vi "cycling structure demo Main.vi"() -> ()   [LabVIEW 2020]
doc: "This VI can be used as a launcher VI for the main application or as a debugging tool.\n_____\nBased on DQMH Project Template 6.1.0.94."
uses:
  Libraries/Rename As Application UI/cycling structure demo UI.lvlib
  Libraries/Launcher Support/Launcher Support.lvlib
  <vilib>/Peloton/Pelobuttons/Pelobuttons_lib_Pelobuttons.lvlib
  <vilib>/Peloton/Peloton Config/DCFG Framework/Peloton_lib_DCFG Framework.lvlib
  Libraries/Rename As Application Shared/Rename as Application Shared.lvlib
panel:
  in  "Config Views":string(combo)
  in  "Launch Peloton Config":bool
  in  "Launch UI API Tester":bool
  out "Command Line Arguments":string[](array[string])
  out "Module Running?":bool
  out "Status":string
  out "error out":errorcluster
  in  "Stop Module":bool
  in  "Start Module":bool
  # "See the Build_Final_EXE bookmarks on the diagram for instructions on using this VI as a launcher for an EXE."
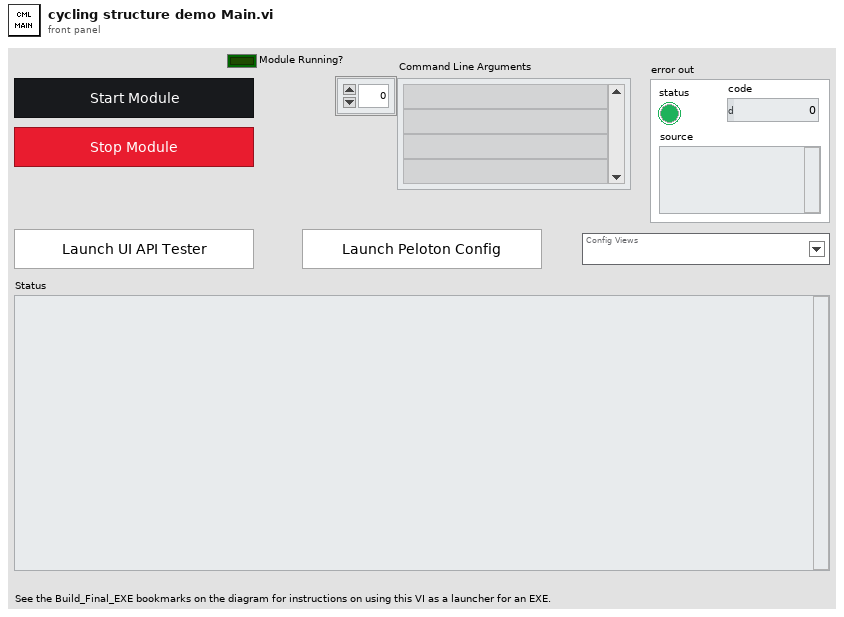
[diagram p1: front panel]
types:
  T1 = typedef "Peloton_lib_DCFG Framework.lvlib/Broadcast Events--cluster.ctl" = cluster{"Module Did Init":refnum<user-event>, "Status Updated":refnum<user-event>, "Error Reported":refnum<user-event>, "Module Did Stop":refnum<user-event>, "Update Module Execution Status":refnum<user-event>, "View Changed":refnum<user-event>, "Main Window Closed":refnum<user-event>, "Configuration Committed":refnum<user-event>, "Configuration Canceled":refnum<user-event>, "Views List Updated":refnum<user-event>, "Config Folder Path Updated":refnum<user-event>}
  T2 = typedef "cycling structure demo UI.lvlib/Broadcast Events--cluster.ctl" = cluster{"Module Did Init":refnum<user-event>, "Status Updated":refnum<user-event>, "Error Reported":refnum<user-event>, "Module Did Stop":refnum<user-event>, "Update Module Execution Status":refnum<user-event>}
  T3 = enum32{"invalid app kind", "Development System", "Run Time System", "Student Edition", "Embedded LabVIEW", "Evaluation", "Custom"}
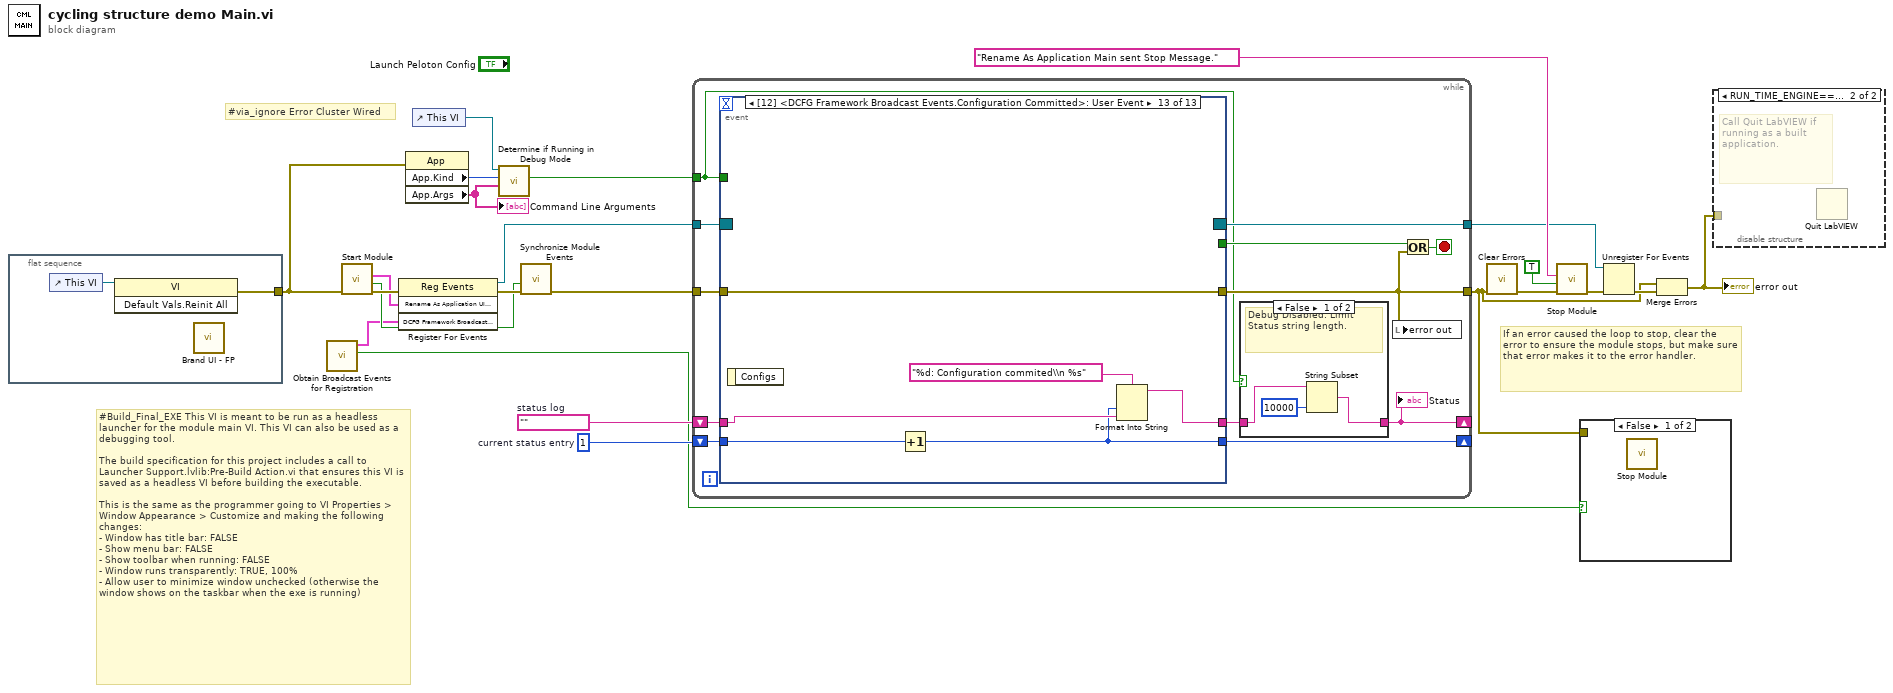
[diagram p0: block diagram]
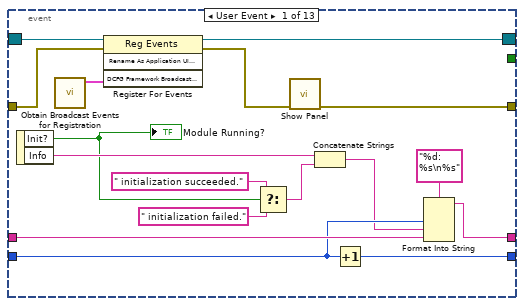
[diagram p4: hidden frame]
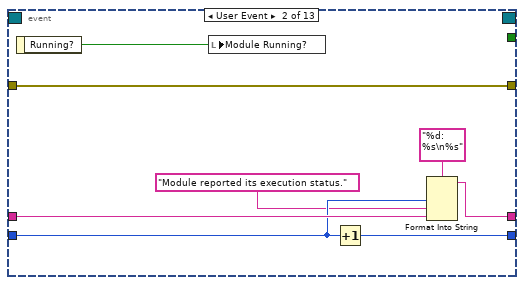
[diagram p5: hidden frame]
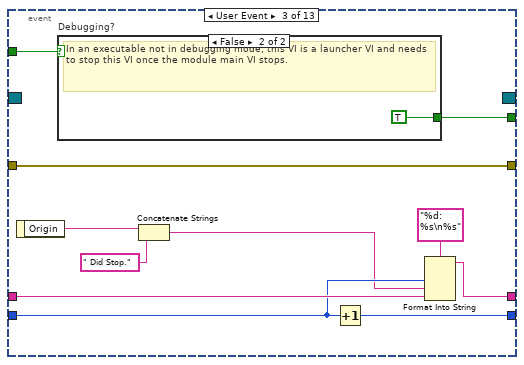
[diagram p6: hidden frame]
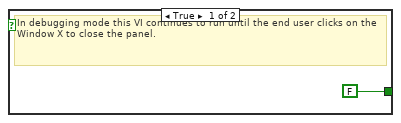
[diagram p7: hidden frame]
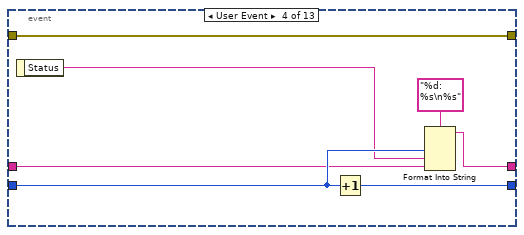
[diagram p8: hidden frame]
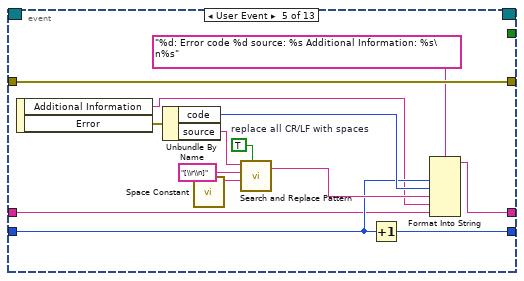
[diagram p9: hidden frame]
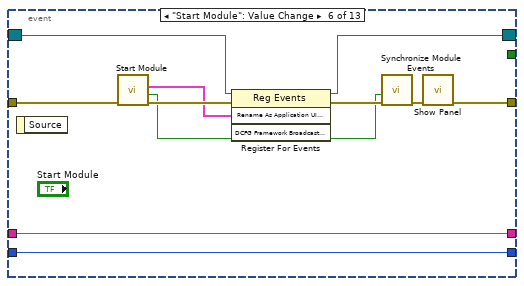
[diagram p10: hidden frame]
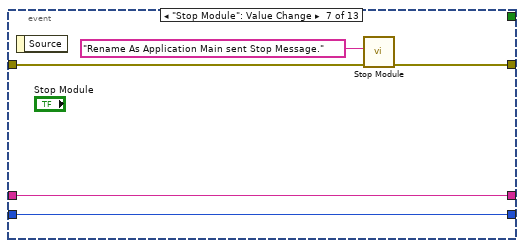
[diagram p11: hidden frame]
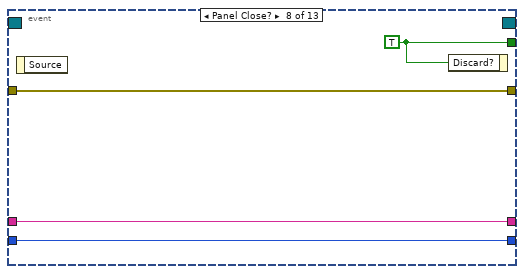
[diagram p12: hidden frame]
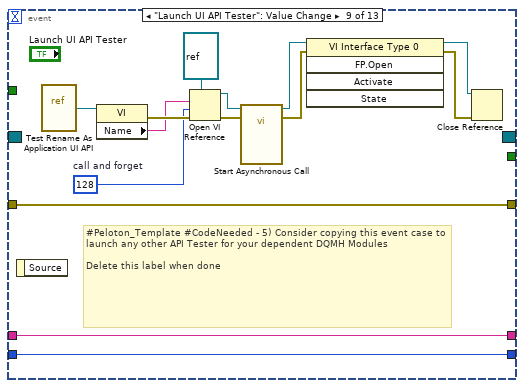
[diagram p13: hidden frame]
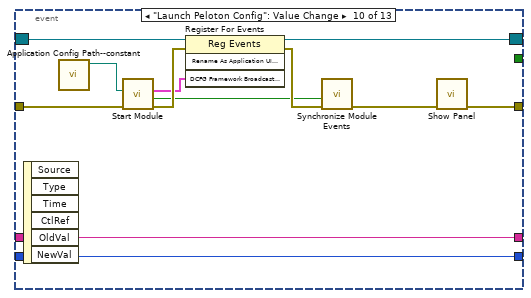
[diagram p14: hidden frame]
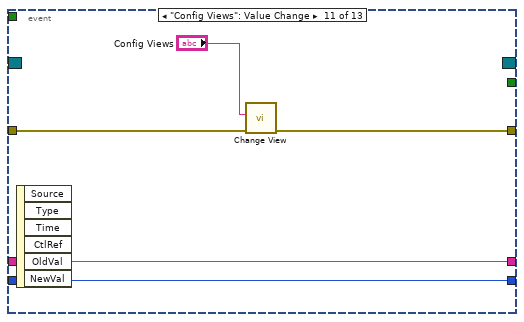
[diagram p15: hidden frame]
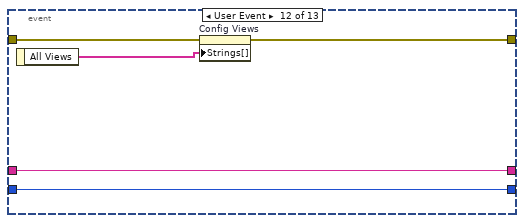
[diagram p16: hidden frame]
diagram:
  w12 = 1  # current status entry
  w13 = ""  # status log
  # "#via_ignore Error Cluster Wired"
  # "#Build_Final_EXE This VI is meant to be run as a headless launcher for the module main VI. This VI can also be used as a debugging tool. \n\nThe build specification for this project includes a call to Launcher Support.lvlib:Pre-Build Action.vi that ensures this VI is saved as a headless VI before building the executable.\n\nThis is the same as the programmer going to VI Properties > Window Appearance > Customize and making the following changes:\n- Window has title bar: FALSE\n- Show menu bar: FALSE\n- Show toolbar when running: FALSE\n- Window runs transparently: TRUE, 100%\n- Allow user to minimize window unchecked (otherwise the window shows on the taskbar when the exe is running)"
  # "If an error caused the loop to stop, clear the error to ensure the module stops, but make sure that error makes it to the error handler."
  n1 = flat-sequence {
    tunnel: [w25] -> w16
    frame #0 {
      n2 = control-ref of="This VI"() -> (w24:refnum<vi>)
      n3 = invoke on="Invoke Node" class="VI" method="Default Vals.Reinit All"(reference=w24) -> (error out=w25:errorcluster)  [unwired: 2 in, 2 out]
      n4 = call <vilib>:"Brand UI - FP.vi"() -> ()  [unwired: 12 in]
    }
  }
  n5 = call <vilib>:"Obtain Broadcast Events for Registration.vi"() -> ("Already running?"=w2:bool, "DCFG Framework Broadcast Events"=w1:T1)  [unwired: 9 in, 1 out]
  n6 = call <vilib>:"Start Module.vi"("error in"=w16) -> ("error out"=w19:errorcluster, "Wait for Event Sync?"=w9:bool, "Rename As Application UI Broadcast Events"=w8:T2)  [unwired: 7 in, 1 out]
  n7 = register-events(error in=w19, w8, w1) -> (reference out=w7:refnum<event-registration>, error out=w20:errorcluster)  [unwired: 1 in]
  n8 = property on="Property Node" class="App"(error in=w16) -> ("App.Kind"=w3:T3, "App.Args"=w6:string[])  [unwired: 1 in, 2 out]
  "Command Line Arguments" <- w6
  n9 = control-ref of="This VI"() -> (w5:refnum<vi>)
  n10 = call "Determine if Running in Debug Mode.vi"("App.Args"=w6, "App.Kind"=w3, "Launcher VI ref"=w5) -> ("Debug mode?"=w4:bool)  [unwired: 8 in]
  n11 = call <vilib>:"Synchronize Module Events.vi"("error in"=w20, "Wait for Event Sync?"=w9) -> ("error out"=w17:errorcluster)  [unwired: 9 in]
  n12 = while {
    tunnel: w7 -> [w35]
    tunnel: [w36] -> w15
    shift-right: [w27] -> _
    shift-left: w13 -> [w32]
    shift-right: [w31] -> _
    shift-left: w12 -> [w33]
    tunnel: w17 -> [w37]
    tunnel: [w29] -> w11
    tunnel: w4 -> [w26]
    stop <- w30 stop-if-true
    n13 = event shown="[12] <DCFG Framework Broadcast Events.Configuration Committed>: User Event" {
      selector: w35 -> [w44 _ _ _ _ w102 _ _ _ w139 _ _ _]
      dyn-events: [w43 _ _ _ _ w101 _ _ _ w138 _ _ _] -> w29
      timeout: _ -> [_ _ _ _ _ _ _ _ _ _ _ _ _]
      tunnel: [_ _ w68 _ _ _ _ w119 _ _ _ _ _] -> w34
      tunnel: [w57 w66 w77 w86 w100 w107 w116 w120 w134 w146 w150 w155 w162] -> w36
      tunnel: w33 -> [w53 w63 w74 w82 w90 w105 w113 w117 w128 w140 w148 w153 w159]
      tunnel: w32 -> [w54 w64 w75 w81 w88 w106 w114 w118 w129 w141 w149 w154 w160]
      tunnel: [w51 w61 w72 w83 w91 w106 w114 w118 w129 w141 w149 w154 w161] -> w28
      tunnel: [w52 w62 w73 w85 w89 w105 w113 w117 w128 w140 w148 w153 w158] -> w31
      tunnel: w37 -> [w58 w66 w77 w86 w100 w109 w115 w120 w134 w143 w151 w156 w162]
      tunnel: w26 -> [_ _ w67 _ _ _ _ _ _ _ _ _ _]
      event User Event {
        n14 = event-data() -> ("Init?"=w48:bool, "Info"=w50:string)  [unwired: 1 in]
        "Module Running?" <- w48
        n15 = call <vilib>:"Obtain Broadcast Events for Registration.vi"() -> ("DCFG Framework Broadcast Events"=w42:T1)  [unwired: 9 in, 2 out]
        n16 = register-events(reference=w44, error in=w58, w42) -> (reference out=w43:refnum<event-registration>, error out=w56:errorcluster)  [unwired: 1 in]
        n17 = Select(t=" initialization succeeded.", s=w48, f=" initialization failed.") -> (s? t:f=w45:string)
        n18 = call <vilib>:"Show Panel.vi"("error in (no error)"=w56) -> ("error out"=w57:errorcluster)  [unwired: 10 in]
        n19 = Concatenate Strings(w50, w45) -> (w49:string)
        n20 = Increment(x=w53) -> (x+1=w52:i32)
        n21 = Format Into String(format string="%d: %s\n%s", w53, w49, w54) -> (resulting string=w51:string)  [unwired: 2 in, 1 out]
      }
      event User Event {
        n22 = event-data() -> ("Running?"=w59:bool)  [unwired: 1 in]
        n23 = local write "Module Running?"(w59) -> ()
        n24 = Increment(x=w63) -> (x+1=w62:i32)
        n25 = Format Into String(format string="%d: %s\n%s", w63, "Module reported its execution status.", w64) -> (resulting string=w61:string)  [unwired: 2 in, 1 out]
      }
      event User Event {
        n26 = event-data() -> ("Origin"=w71:string)  [unwired: 1 in]
        n27 = case "Debugging?" shown="False" w67 {
          tunnel: [FALSE ("Discard?") TRUE ("Discard?")] -> w68
          frame True {
            # "In debugging mode this VI continues to run until the end user clicks on the Window X to close the panel."
          }
          frame False {
            # "In an executable not in debugging mode, this VI is a launcher VI and needs to stop this VI once the module main VI stops."
          }
        }
        n28 = Concatenate Strings(w71, " Did Stop.") -> (w70:string)
        n29 = Increment(x=w74) -> (x+1=w73:i32)
        n30 = Format Into String(format string="%d: %s\n%s", w74, w70, w75) -> (resulting string=w72:string)  [unwired: 2 in, 1 out]
      }
      event User Event {
        n31 = event-data() -> ("Status"=w80:string)  [unwired: 1 in]
        n32 = Increment(x=w82) -> (x+1=w85:i32)
        n33 = Format Into String(format string="%d: %s\n%s", w82, w80, w81) -> (resulting string=w83:string)  [unwired: 2 in, 1 out]
      }
      event User Event {
        w95 = TRUE  # replace all CR/LF with spaces
        n34 = event-data() -> ("Additional Information"=w87:string, "Error"=w99:errorcluster)  [unwired: 1 in]
        n35 = Unbundle By Name(w99) -> ("code"=w92:i32, "source"=w93:string)
        n36 = call <vilib>:"Space Constant.vi"() -> ("String"=w96:string)
        n37 = call <vilib>:"Search and Replace Pattern.vi"("string"=w93, "regular expression (\"\")"="[\\r\\n]" ("regular expression (\"\")"), "replace string (\"\")"=w96, "replace all? (F)"=w95) -> ("result string"=w94:string)  [unwired: 1 in, 1 out]
        n38 = Increment(x=w90) -> (x+1=w89:i32)
        n39 = Format Into String(format string="%d: Error code %d source: %s Additional Information: %s\n%s", w90, w92, w94, w87, w88) -> (resulting string=w91:string)  [unwired: 2 in, 1 out]
      }
      event "Start Module": Value Change {
        n40 = event-data() -> ()  [unwired: 1 in, 1 out]
        n41 = call <vilib>:"Start Module.vi"("error in"=w109) -> ("error out"=w110:errorcluster, "Wait for Event Sync?"=w104:bool, "Rename As Application UI Broadcast Events"=w103:T2)  [unwired: 7 in, 1 out]
        n42 = register-events(reference=w102, error in=w110, w103) -> (reference out=w101:refnum<event-registration>, error out=w111:errorcluster)  [unwired: 1 in]
        n43 = call <vilib>:"Synchronize Module Events.vi"("error in"=w111, "Wait for Event Sync?"=w104) -> ("error out"=w108:errorcluster)  [unwired: 9 in]
        n44 = call <vilib>:"Show Panel.vi"("error in (no error)"=w108) -> ("error out"=w107:errorcluster)  [unwired: 10 in]
      }
      event "Stop Module": Value Change {
        n45 = event-data() -> ()  [unwired: 1 in, 1 out]
        n46 = call <vilib>:"Stop Module.vi"("error in"=w115, "Origin"="Rename As Application Main sent Stop Message.") -> ("error out"=w116:errorcluster)  [unwired: 9 in]
      }
      event Panel Close? {
        w119 = TRUE ("Discard?")
        n47 = event-data() -> ()  [unwired: 1 in, 1 out]
        n48 = event-data ("Event Filter Node")("Discard?"=w119) -> ()  [unwired: 1 in, 1 out]
      }
      event "Launch UI API Tester": Value Change {
        w123 = 128  # call and forget
        # "#Peloton_Template #CodeNeeded - 5) Consider copying this event case to launch any other API Tester for your dependent DQMH Modules\n\nDelete this label when done"
        n49 = event-data() -> ()  [unwired: 1 in, 1 out]
        n50 = vi-ref "Test Rename As Application UI API.vi"() -> (w126:refnum<vi>)
        n51 = property class="VI"(reference=w126) -> (error out=w133:errorcluster, "Name"=w127:string)  [unwired: 1 in, 1 out]
        n52 = Open VI Reference(type specifier VI Refnum (for type only)=refnum<vi> refnum, vi path=w127, options=w123, error in (no error)=w133) -> (vi reference=w125:refnum<vi>, error out=w132:errorcluster)  [unwired: 2 in]
        n53 = call-by-ref "Start Asynchronous Call"(reference=w125, error in=w132) -> (reference out=w122:refnum<vi>, error out=w131:errorcluster)  [unwired: 12 in]
        n54 = invoke class="VI Interface Type 0" method="FP.Open"(reference=w122, error in=w131) -> (reference out=w121:refnum<vi>, error out=w130:errorcluster)  [unwired: 3 in, 3 out]
        n55 = Close Reference(reference=w121, error in (no error)=w130) -> ()  [unwired: 1 out]
      }
      event "Launch Peloton Config": Value Change {
        n56 = event-data() -> ()  [unwired: 1 in, 6 out]
        n57 = call "Application Config Path--constant.vi"() -> ("File Path"=w135:path)  [unwired: 11 in]
        n58 = call <vilib>:"Start Module.vi"("error in"=w143, "Config Folder"=w135) -> ("error out"=w142:errorcluster, "Wait for Event Sync?"=w136:bool, "DCFG Framework Broadcast Events"=w137:T1)  [unwired: 6 in, 1 out]
        n59 = register-events(reference=w139, error in=w142, w137) -> (reference out=w138:refnum<event-registration>, error out=w145:errorcluster)  [unwired: 1 in]
        n60 = call <vilib>:"Synchronize Module Events.vi"("error in (no error)"=w145, "Wait for Event Sync?"=w136) -> ("error out"=w144:errorcluster)  [unwired: 9 in]
        n61 = call <vilib>:"Show Panel.vi"("error in"=w144) -> ("error out"=w146:errorcluster)  [unwired: 10 in]
      }
      event "Config Views": Value Change {
        n62 = event-data() -> ()  [unwired: 1 in, 6 out]
        n63 = call <vilib>:"Change View.vi"("error in"=w151, "View"="Config Views") -> ("error out"=w150:errorcluster)  [unwired: 9 in]
      }
      event User Event {
        n64 = event-data() -> ("All Views"=w152:string[])  [unwired: 1 in]
        n65 = property on="Config Views" class="CmbBox"(error in=w156, "Strings[]"=w152) -> (error out=w155:errorcluster)  [unwired: 1 in, 1 out]
      }
      event User Event {
        n66 = event-data() -> ()  [unwired: 1 in, 1 out]
        n67 = Increment(x=w159) -> (x+1=w158:i32)
        n68 = Format Into String(format string="%d: Configuration commited\\n %s", w158, w160) -> (resulting string=w161:string)  [unwired: 2 in, 1 out]
      }
    }
    n69 = case shown="False" w26 {
      tunnel: w28 -> [w40 w41]
      tunnel: [w38 w41] -> w27
      frame False {
        # "Debug Disabled. Limit Status string length."
        n70 = String Subset(string=w40, length (rest)=10000 ("length (rest)")) -> (substring=w38:string)  [unwired: 1 in]
      }
      frame True {
        # "Debug Eneabled. Do not limit Status string length."
      }
    }
    "Status" <- w27
    n71 = local write "error out"(w36) -> ()
    n72 = Or(x=w34, y=w36) -> (x .or. y?=w30:bool)
  }
  n73 = call <vilib>:"Clear Errors.vi"("error in (no error)"=w15) -> ("error out"=w21:errorcluster)  [unwired: 5 in, 1 out]
  n74 = call <vilib>:"Stop Module.vi"("error in"=w21, "Wait for Module to Stop? (F)"=TRUE ("Wait for Module to stop?"), "Origin"="Rename As Application Main sent Stop Message.") -> ("error out"=w22:errorcluster)  [unwired: 8 in]
  n75 = case shown="False" w2 {
    tunnel: w15 -> [_ _]
    frame False {
      n76 = call <vilib>:"Stop Module.vi"() -> ()  [unwired: 11 in, 1 out]
    }
    frame True {
    }
  }
  n77 = Unregister For Events(event registration refnum=w11, error in=w22) -> (error out=w23:errorcluster)
  n78 = Merge Errors(w15, w23) -> (w18:errorcluster)
  "error out" <- w18
  n79 = disable-structure "Conditional Disable Structure" shown="RUN_TIME_ENGINE==True" {
    disable-tunnel: w18 -> [_ _]
    frame condition #0 (active) {
    }
    frame condition #1 {
      # "Call Quit LabVIEW if running as a built application."
      n80 = Quit LabVIEW() -> ()  [unwired: 1 in]
    }
  }
